vi "Initialize - Test.vi"() -> ()   [LabVIEW 2017]
panel:
  out "error out":errorcluster
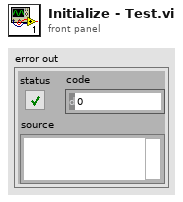
[diagram p1: front panel]
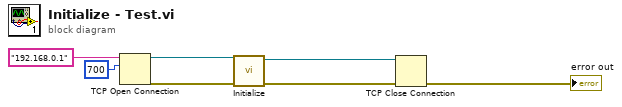
[diagram p0: block diagram]
diagram:
  n1 = TCP Open Connection(address="192.168.0.1", remote port or service name=u16 700) -> (connection ID=w5:refnum<k5>, error out=w4:errorcluster)  [unwired: 3 in]
  n2 = call "Initialize.vi"("error in (no error)"=w4, "TCP Network Connection in"=w5) -> ("error out"=w2:errorcluster, "TCP Network Connection out"=w3:refnum<k5>)  [unwired: 6 in, 2 out]
  n3 = TCP Close Connection(connection ID=w3, error in (no error)=w2) -> (error out=→"error out":errorcluster)  [unwired: 1 in, 1 out]
